vi "Retrieve Block Data Refs from item refs (outgoing).vi"(8 "error in":errorcluster, 10 "inline vs group data refs":T3 {"item refs - status" format="%.0x"; "item refs - data" format="%.0x"}, 11 "Section Ref in":T4 format="%.0x") -> (0 "error out":errorcluster, 1 "Block Data Refs - data":T1[](array[typedef]) {"Data Reference" format="%.0x"}, 2 "Block Data Refs - status":T1[](array[typedef]) {"Data Reference" format="%.0x"}, 3 "Device Ref out":T4 format="%.0x", 4 "size - data":i32, 5 "size - info":i32)   [LabVIEW 2019, in "HLA Custom Device System Explorer.lvlib"]
uses:
  HLA Custom Device System Explorer.lvlib
  <vilib>/NI VeriStand/Custom Device API/Block Data Reference.ctl
  <vilib>/NI VeriStand/Custom Device API/Data Reference.ctl
  <vilib>/NI VeriStand/Custom Device API/Custom Device Item Ref.ctl
  Shared/inline_vs_group_refs.ctl
  <vilib>/NI VeriStand/Custom Device API/Data Access Type.ctl
  <vilib>/NI VeriStand/Custom Device API/Custom Device API.lvlib
  Shared/HLA Custom Device Shared.lvlib
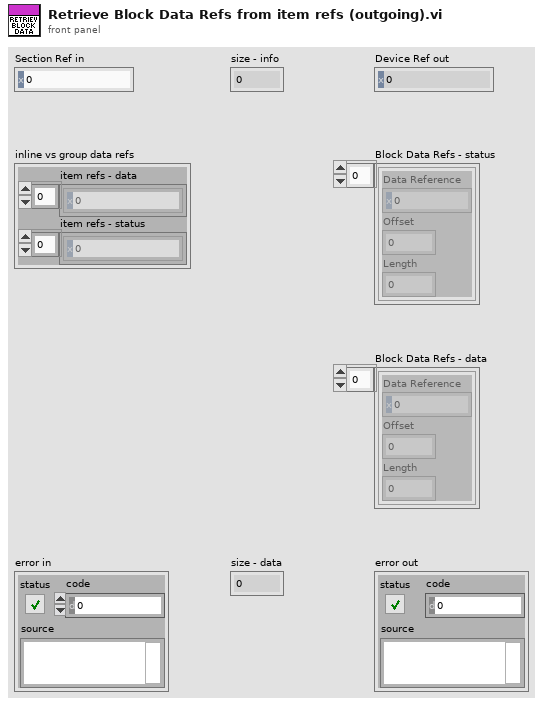
[diagram p1: front panel]
types:
  T1 = typedef "Custom Device API.lvlib/Block Data Reference.ctl" = cluster{"Data Reference":T2, "Offset":u64, "Length":u64}
  T2 = typedef "Custom Device API.lvlib/Data Reference.ctl" = i32
  T3 = typedef "HLA Custom Device Shared.lvlib/inline_vs_group_refs.ctl" = cluster{"item refs - data":T4[], "item refs - status":T4[]}
  T4 = typedef "Custom Device API.lvlib/Custom Device Item Ref.ctl" = u64
  T5 = typedef "Custom Device API.lvlib/Data Access Type.ctl" = enum16{"Read", "Write"}
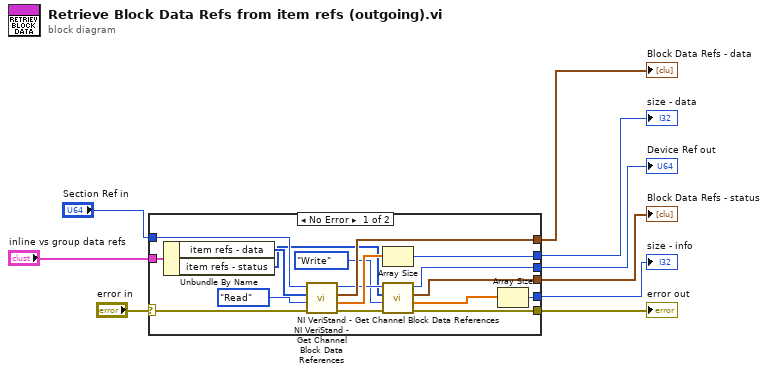
[diagram p0: block diagram]
diagram:
  n1 = case shown="No Error" "error in" {
    selector: "error in" -> [w21 w28]
    tunnel: [w26 _] -> w3
    tunnel: [w25 _] -> w4
    tunnel: [w18 w27] -> w9
    tunnel: [w13 w28] -> w8
    tunnel: "Section Ref in" -> [w22 w27]
    tunnel: "inline vs group data refs" -> [w20 _]
    tunnel: [w16 _] -> w2
    tunnel: [w15 _] -> w1
    frame No Error {
      n2 = Unbundle By Name(w20) -> ("item refs - data"=w12:T4[], "item refs - status"=w11:T4[])
      n3 = call <vilib>:"NI VeriStand - Get Channel Block Data References.vi"("error in (no error)"=w21, "Access"=Data_Access_Type."Read", "Channel Refs"=w12, "Device Ref in"=w22) -> ("error out"=w14:errorcluster, "Values Array"=w24:dbl[], "Block Data Refs"=w25:T1[], "Device Ref out"=w19:T4)  [unwired: 4 in]
      n4 = Array Size(array=w24) -> (size(s)=w26:i32)
      n5 = call <vilib>:"NI VeriStand - Get Channel Block Data References.vi"("error in (no error)"=w14, "Access"=Data_Access_Type."Write", "Channel Refs"=w11, "Device Ref in"=w19) -> ("error out"=w13:errorcluster, "Values Array"=w17:dbl[], "Block Data Refs"=w15:T1[], "Device Ref out"=w18:T4)  [unwired: 4 in]
      n6 = Array Size(array=w17) -> (size(s)=w16:i32)
    }
    frame Error {
    }
  }
  "size - info" <- w2
  "Block Data Refs - status" <- w1
  "Device Ref out" <- w9
  "error out" <- w8
  "Block Data Refs - data" <- w4
  "size - data" <- w3
